vi "ViChoice.vi"() -> ()   [LabVIEW 2015]
uses:
  GlobalPath.vi
  GlobalVi.vi
  GlobalData.vi
panel:
  out "Finalization":bool
  out "Lines":string[](array[string])
  out "PinInsertGlue":bool
  out "QAQCvacoff":bool
  out "StiffRemoval":bool
  out "QAQCvacon":bool
  out "DrunRunFull":bool
  out "AllCoolBar":bool
  out "AddHoneycomb":bool
  out "AddFrame":bool
  out "PCBalignStiff":bool
  out "PCBposStiff":bool
  out "PCBalignTab":bool
  out "NewPanel":bool
  in  "Construction Finalization":bool
  in  "Panel QA/QC vacuum off":bool
  in  "Gluing of alignment pin/insert":bool
  in  "Panel QA/QC vacuum on":bool
  in  "Stiffback removal":bool
  in  "Add Cooling Bars":bool
  in  "Add Honeycomb":bool
  in  "Add Frames":bool
  in  "Dry Run (full)":bool
  in  "PCB Alignment on stiffback":bool
  in  "PCB Positioning on stiffback":bool
  in  "PCB Alignment on table":bool
  in  "New Panel":bool
  in  "current vi path":path
  out "Opening program":string
  in  "PCB gluing on table":bool
  in  "Internal structure positioning":bool
  in  "Stiffback gluing":bool
  in  "PCB Positioning on table":bool
  in  "Panel Closure":bool
  out "closePanel":bool
  out "PCBposTab":bool
  out "stbackPCBglue":bool
  out "tablePCBglue":bool
  out "innerStructure":bool
  # "Status"
  # "Control"
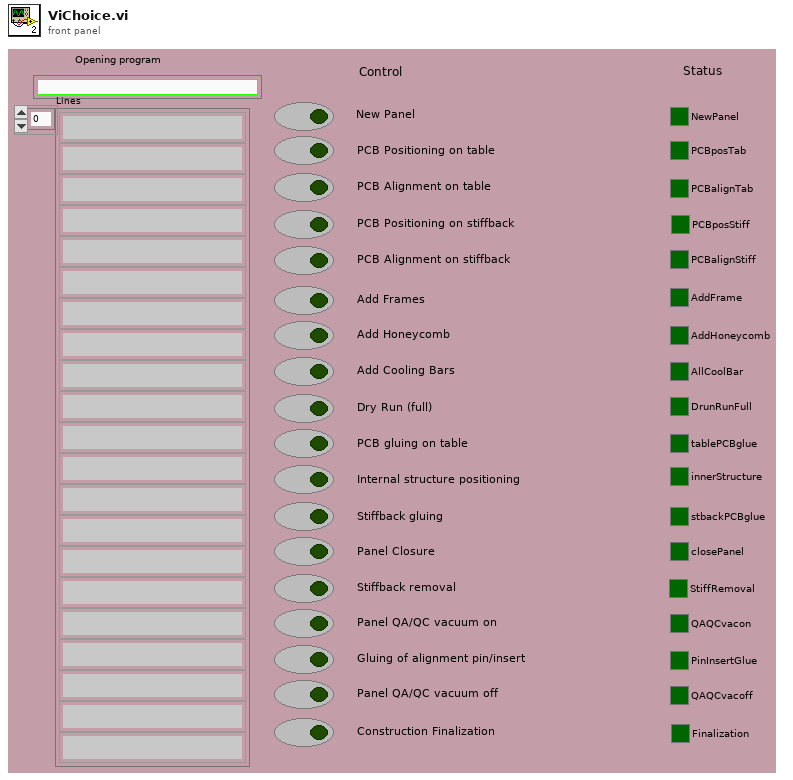
[diagram p1: front panel]
types:
  T1 = enum16{"open", "replace", "create", "open or create", "replace or create", "replace or create with confirmation"}
  T2 = cluster{"top":i32, "left":i32, "bottom":i32, "right":i32}
  T3 = enum32{"Bad", "Idle", "Run top level", "Running"}
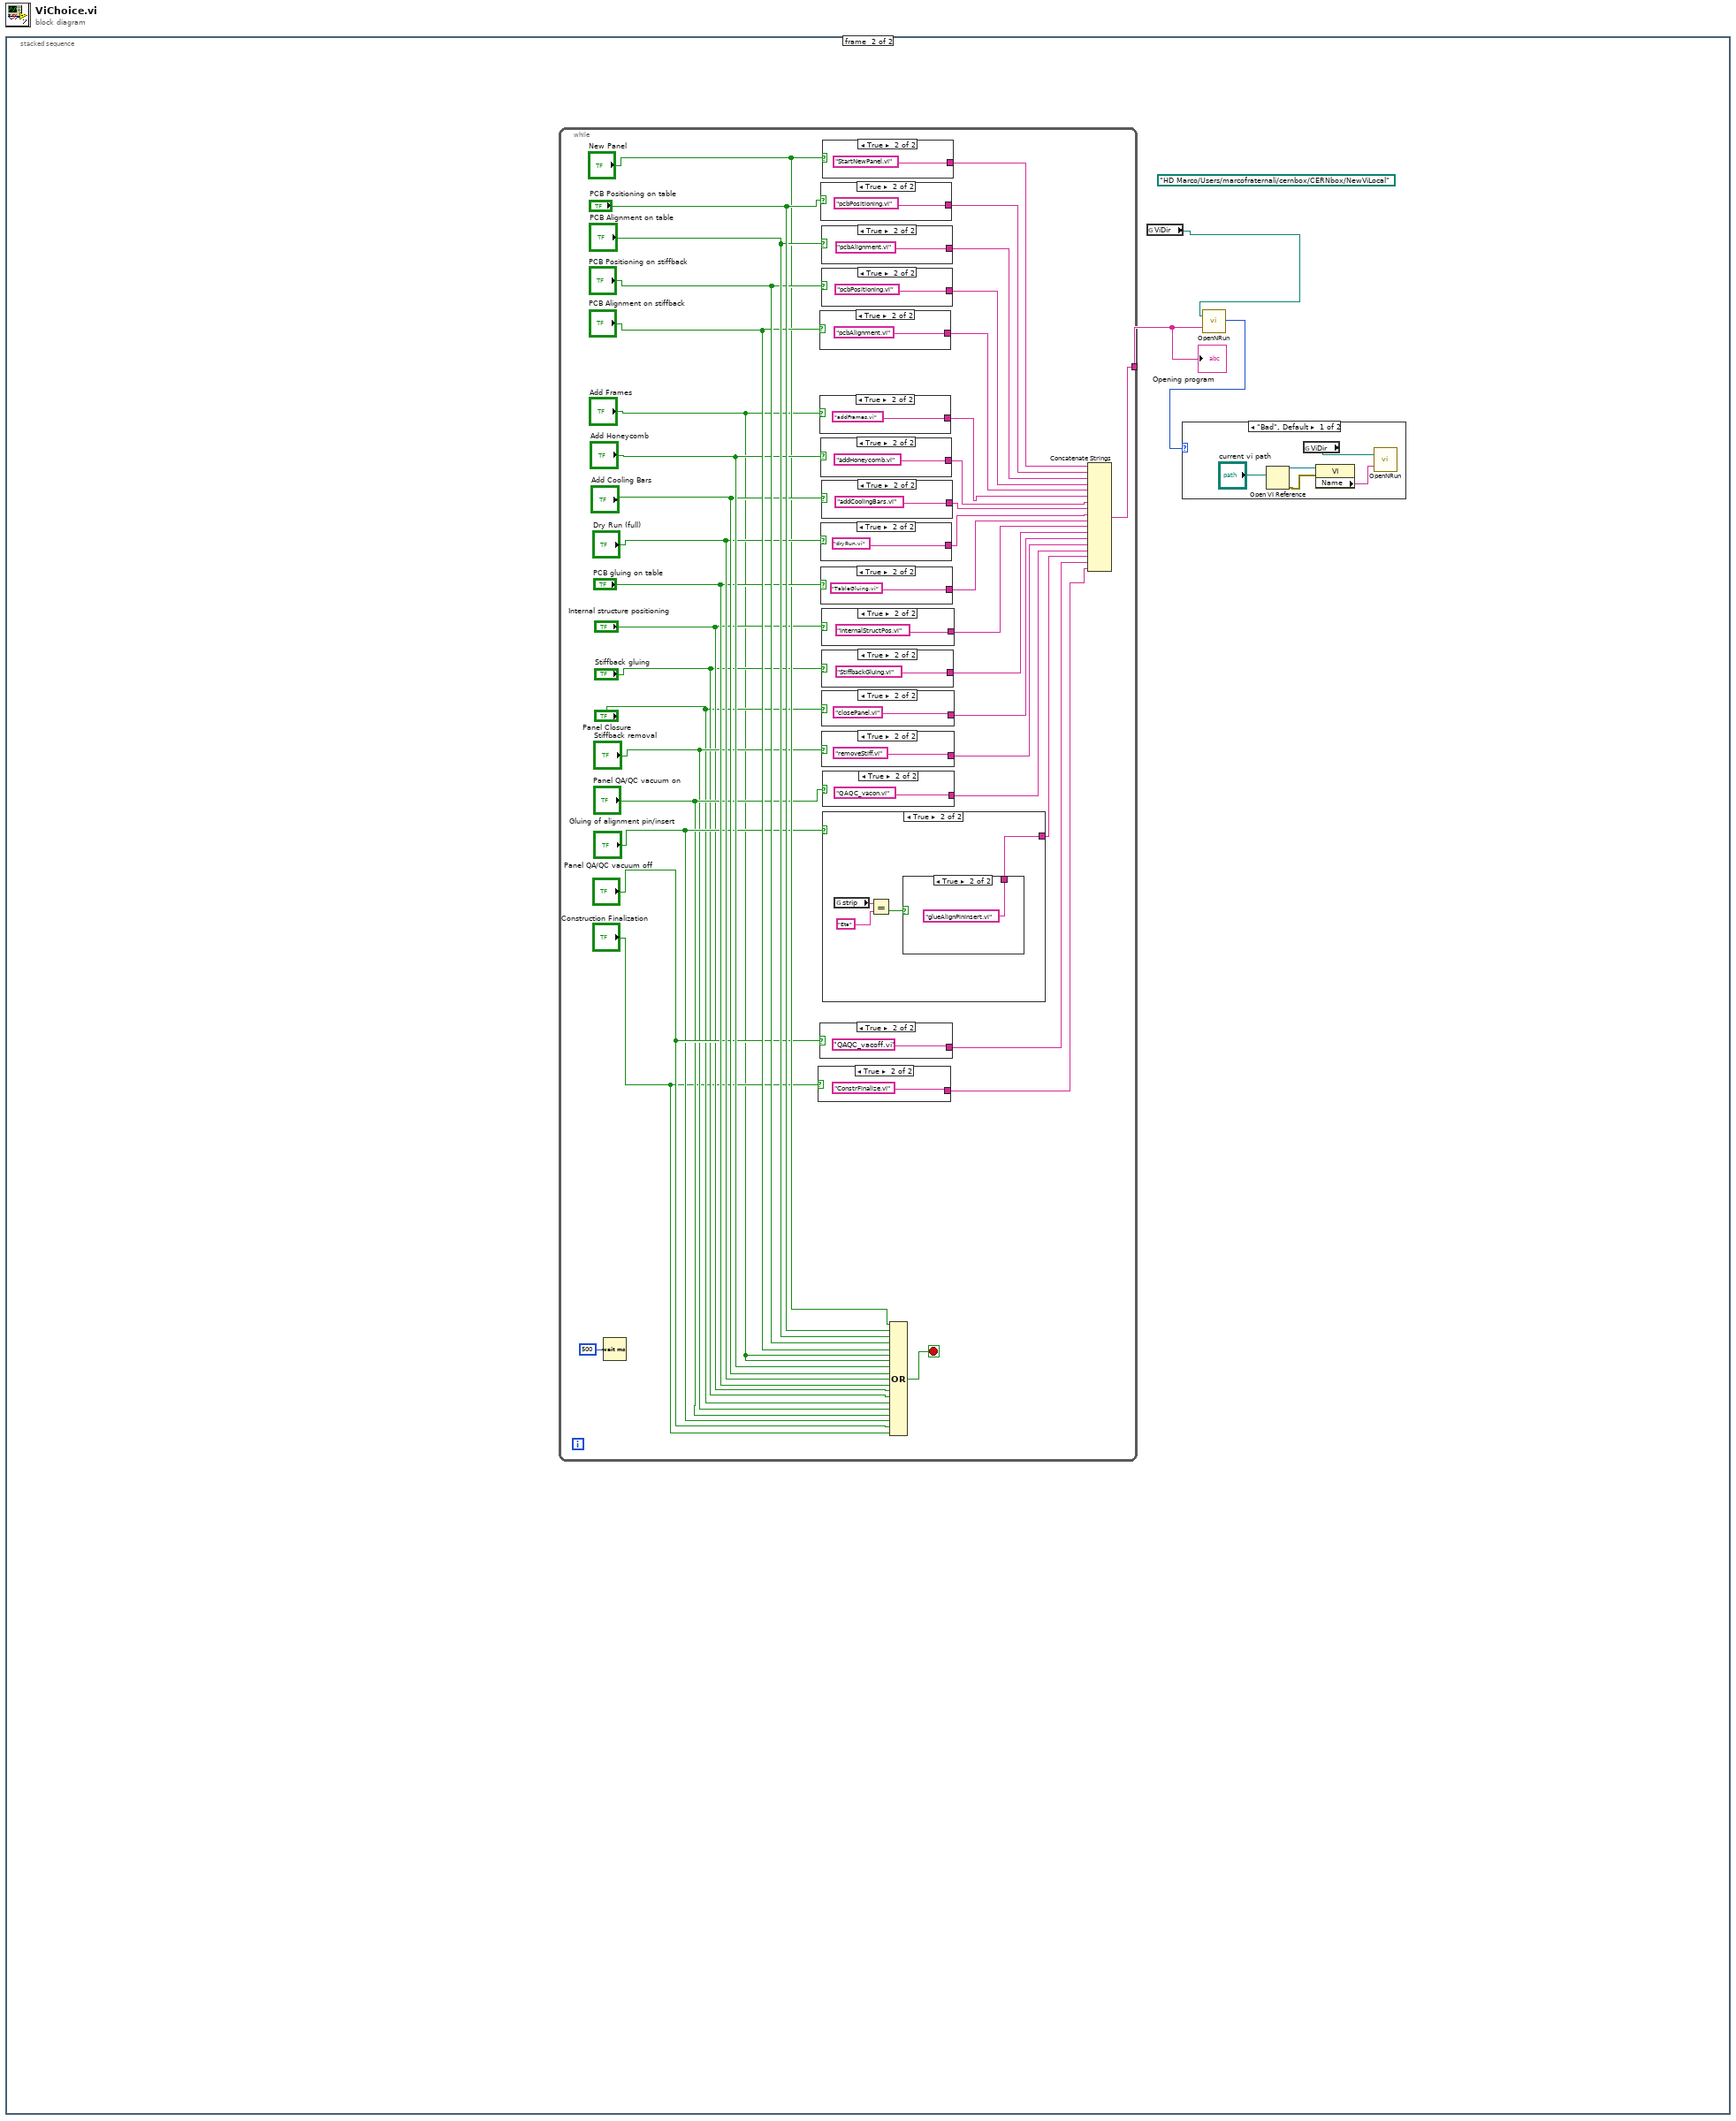
[diagram p0: block diagram]
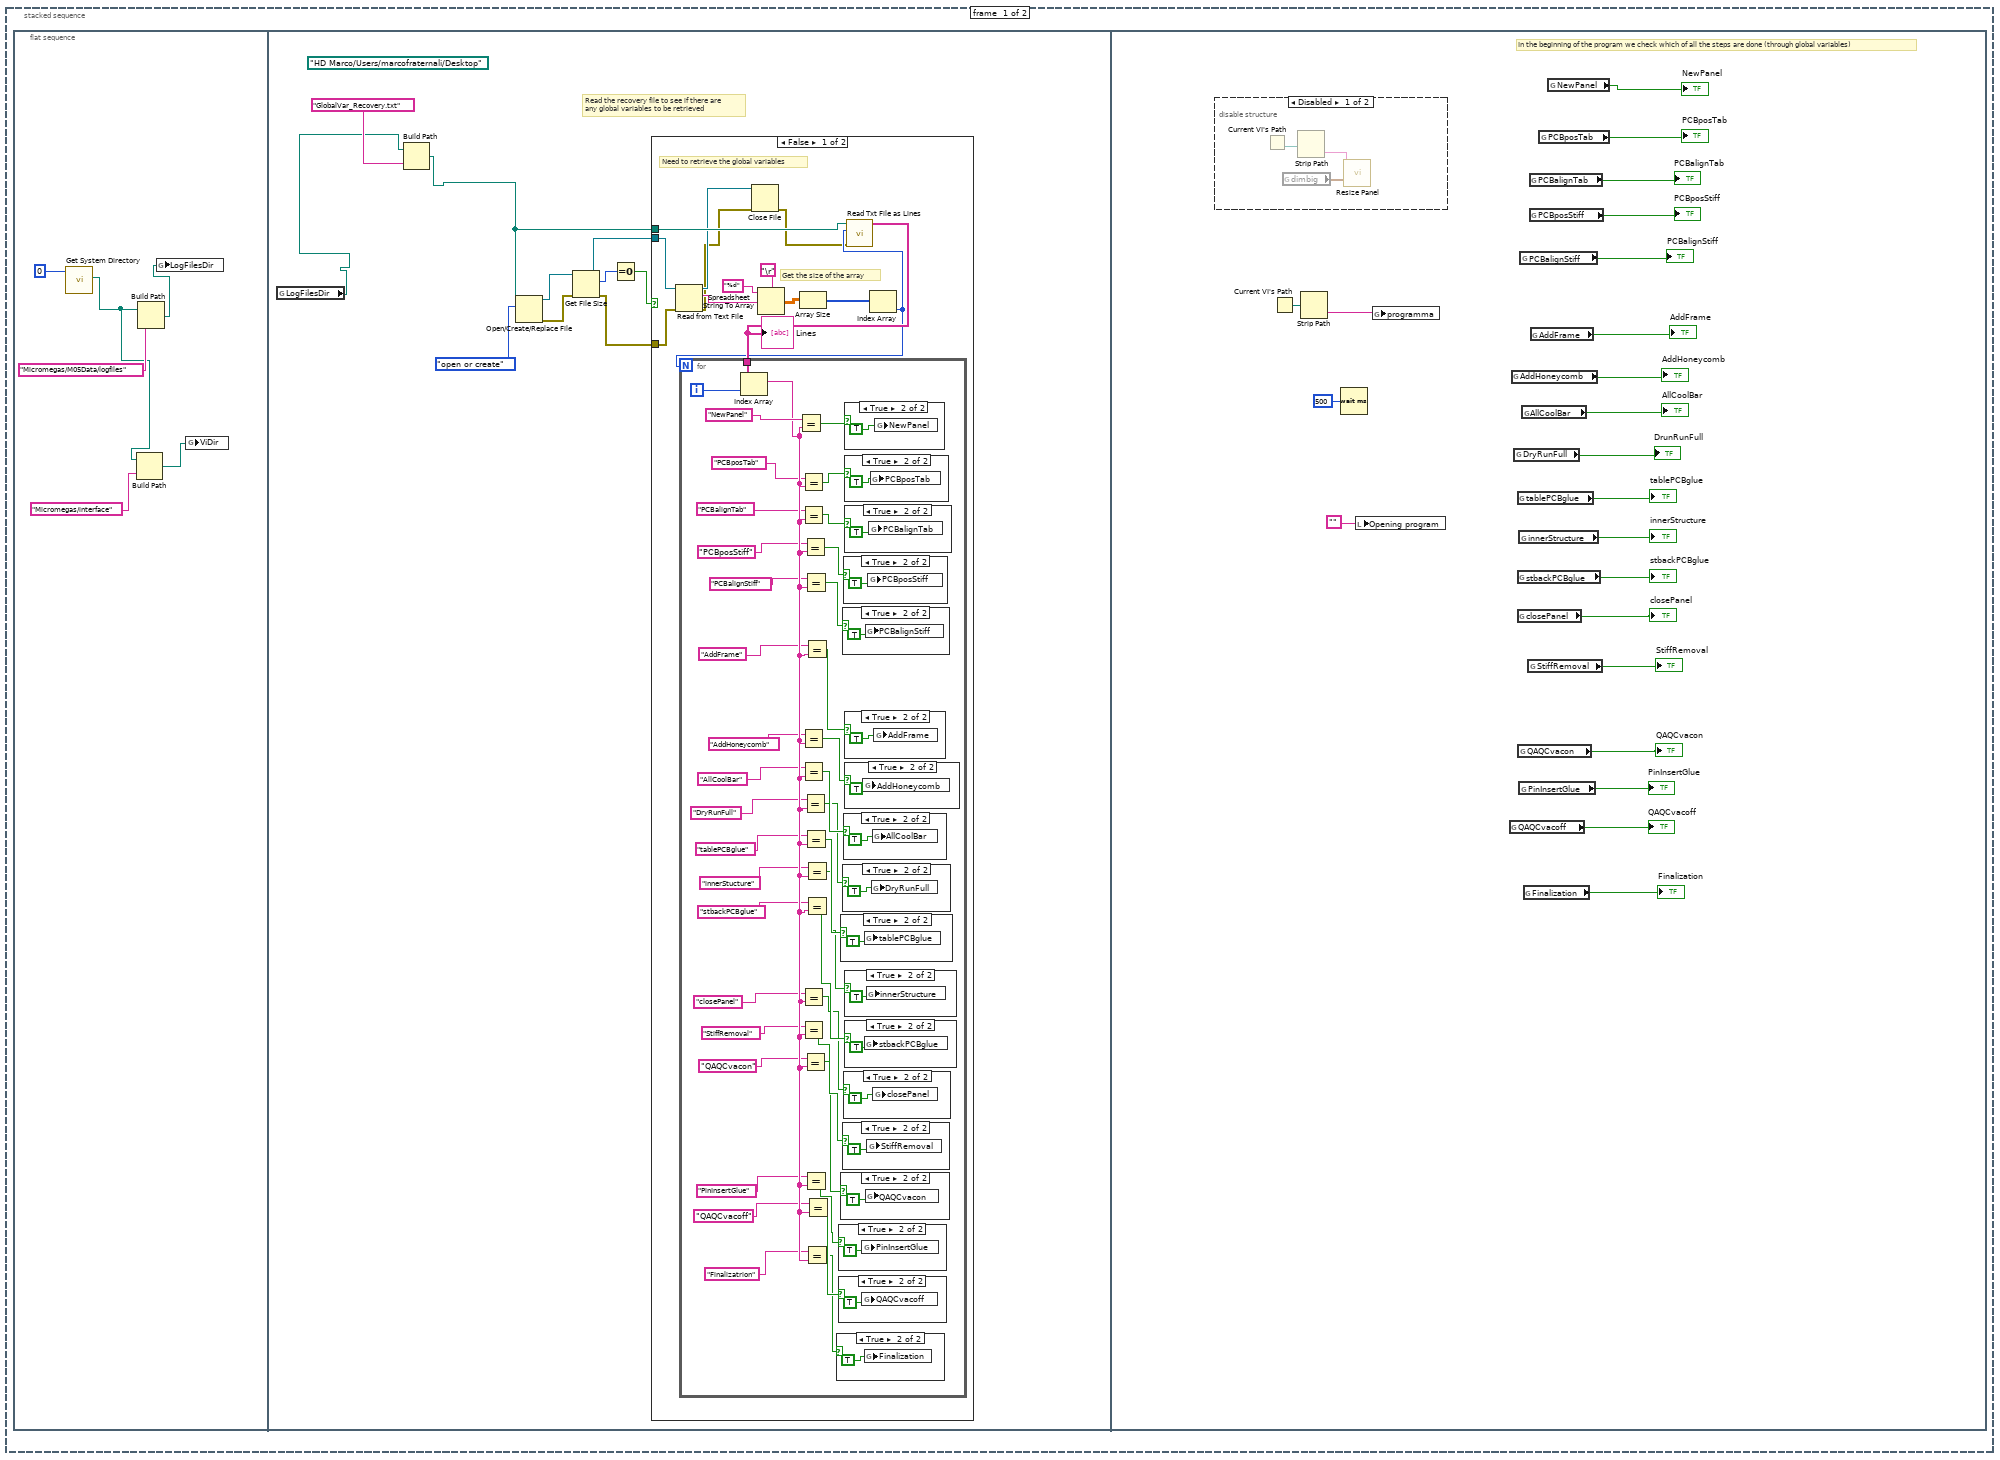
[diagram p2: hidden frame]
diagram:
  n1 = stacked-sequence {
    frame #0 {
      n2 = flat-sequence {
        frame #0 {
          n3 = call <vilib>:"Get System Directory.vi"("system directory type"=0) -> ("system directory"=w3:path)  [unwired: 10 in]
          n4 = Build Path(base path=w3, name or relative path="Micromegas/interface") -> (appended path=w2:path)
          n5 = Build Path(base path=w3, name or relative path="Micromegas/M05Data/logfiles") -> (appended path=w4:path)
          n6 = global write "GlobalPath.vi" "LogFilesDir"(w4) -> ()
          n7 = global write "GlobalPath.vi" "ViDir"(w2) -> ()
        }
        frame #1 {
          (unwired) path "/HD Marco/Users/marcofraternali/Desktop" ("path")
          # "Read the recovery file to see if there are\nany global variables to be retrieved"
          n8 = global read "GlobalPath.vi" "LogFilesDir"() -> (w7:path)
          n9 = Build Path(base path=w7, name or relative path="GlobalVar_Recovery.txt") -> (appended path=w8:path)
          n10 = Open/Create/Replace File(file path (use dialog)=w8, operation (0:open)=T1."open or create") -> (refnum out=w15:refnum<file>, error out=w13:errorcluster)  [unwired: 4 in, 1 out]
          n11 = Get File Size(file=w15, error in=w13) -> (refnum out=w11:refnum<file>, size (in bytes)=w14:i64, 0:w10:errorcluster)
          n12 = Equal To 0?(x=w14) -> (x = 0?=w12:bool)
          n13 = case shown="False" w12 {
            tunnel: w11 -> [w24 _]
            tunnel: w10 -> [w26 _]
            tunnel: w8 -> [w23 _]
            frame False {
              # "Get the size of the array"
              # "Need to retrieve the global variables"
              n14 = Read from Text File(file (use dialog)=w24, error in=w26) -> (refnum out=w19:refnum<file>, text=w27:string, error out=w18:errorcluster)  [unwired: 3 out]
              n15 = Close File(refnum=w19, error in=w18) -> (error out=w17:errorcluster)  [unwired: 1 out]
              n16 = Spreadsheet String To Array(delimiter (Tab)="\r", format string="%d", spreadsheet string=w27) -> (array=w25:dbl[][])  [unwired: 1 out]
              n17 = Array Size(array=w25) -> (size(s)=w22:i32[])
              n18 = Index Array(array=w22) -> (element=w20:i32)  [unwired: 1 in]
              n19 = call "Read Txt File as Lines.vi"("error in"=w17, "Lines to Read"=w20, "file path (use dialog)"=w23) -> ("Lines"=w21:string[])  [unwired: 7 in, 1 out]
              "Lines" <- w21
              n20 = for {
                N: w20 -> [_]
                tunnel: w21 -> [w68]
                i -> [w32]
                n21 = Index Array(array=w68, index=w32) -> (element=w49:string)
                n22 = Equal?(x="NewPanel", y=w49) -> (x = y?=w67:bool)
                n23 = Equal?(x="PCBposTab", y=w49) -> (x = y?=w66:bool)
                n24 = Equal?(x="PCBalignTab", y=w49) -> (x = y?=w65:bool)
                n25 = Equal?(x="AddHoneycomb", y=w49) -> (x = y?=w61:bool)
                n26 = Equal?(x="AllCoolBar", y=w49) -> (x = y?=w60:bool)
                n27 = Equal?(x="closePanel", y=w49) -> (x = y?=w55:bool)
                n28 = Equal?(x="StiffRemoval", y=w49) -> (x = y?=w54:bool)
                n29 = Equal?(x="PCBposStiff", y=w49) -> (x = y?=w64:bool)
                n30 = Equal?(x="DryRunFull", y=w49) -> (x = y?=w59:bool)
                n31 = Equal?(x="QAQCvacon", y=w49) -> (x = y?=w53:bool)
                n32 = Equal?(x="PCBalignStiff", y=w49) -> (x = y?=w63:bool)
                n33 = Equal?(x="tablePCBglue", y=w49) -> (x = y?=w58:bool)
                n34 = Equal?(x="PinInsertGlue", y=w49) -> (x = y?=w52:bool)
                n35 = Equal?(x="AddFrame", y=w49) -> (x = y?=w62:bool)
                n36 = Equal?(x="innerStucture", y=w49) -> (x = y?=w57:bool)
                n37 = Equal?(x="stbackPCBglue", y=w49) -> (x = y?=w56:bool)
                n38 = Equal?(x="Finalizatrion", y=w49) -> (x = y?=w30:bool)
                n39 = Equal?(x="QAQCvacoff", y=w49) -> (x = y?=w51:bool)
                n40 = case shown="True" w30 {
                  frame False {
                  }
                  frame True {
                    n41 = global write "GlobalVi.vi" "Finalization"(TRUE) -> ()
                  }
                }
                n42 = case shown="True" w52 {
                  frame False {
                  }
                  frame True {
                    n43 = global write "GlobalVi.vi" "PinInsertGlue"(TRUE) -> ()
                  }
                }
                n44 = case shown="True" w51 {
                  frame False {
                  }
                  frame True {
                    n45 = global write "GlobalVi.vi" "QAQCvacoff"(TRUE) -> ()
                  }
                }
                n46 = case shown="True" w58 {
                  frame False {
                  }
                  frame True {
                    n47 = global write "GlobalVi.vi" "tablePCBglue"(TRUE) -> ()
                  }
                }
                n48 = case shown="True" w53 {
                  frame False {
                  }
                  frame True {
                    n49 = global write "GlobalVi.vi" "QAQCvacon"(TRUE) -> ()
                  }
                }
                n50 = case shown="True" w63 {
                  frame False {
                  }
                  frame True {
                    n51 = global write "GlobalVi.vi" "PCBalignStiff"(TRUE) -> ()
                  }
                }
                n52 = case shown="True" w59 {
                  frame False {
                  }
                  frame True {
                    n53 = global write "GlobalVi.vi" "DryRunFull"(TRUE) -> ()
                  }
                }
                n54 = case shown="True" w54 {
                  frame False {
                  }
                  frame True {
                    n55 = global write "GlobalVi.vi" "StiffRemoval"(TRUE) -> ()
                  }
                }
                n56 = case shown="True" w64 {
                  frame False {
                  }
                  frame True {
                    n57 = global write "GlobalVi.vi" "PCBposStiff"(TRUE) -> ()
                  }
                }
                n58 = case shown="True" w60 {
                  frame False {
                  }
                  frame True {
                    n59 = global write "GlobalVi.vi" "AllCoolBar"(TRUE) -> ()
                  }
                }
                n60 = case shown="True" w55 {
                  frame False {
                  }
                  frame True {
                    n61 = global write "GlobalVi.vi" "closePanel"(TRUE) -> ()
                  }
                }
                n62 = case shown="True" w67 {
                  frame False {
                  }
                  frame True {
                    n63 = global write "GlobalVi.vi" "NewPanel"(TRUE) -> ()
                  }
                }
                n64 = case shown="True" w66 {
                  frame False {
                  }
                  frame True {
                    n65 = global write "GlobalVi.vi" "PCBposTab"(TRUE) -> ()
                  }
                }
                n66 = case shown="True" w65 {
                  frame False {
                  }
                  frame True {
                    n67 = global write "GlobalVi.vi" "PCBalignTab"(TRUE) -> ()
                  }
                }
                n68 = case shown="True" w62 {
                  frame False {
                  }
                  frame True {
                    n69 = global write "GlobalVi.vi" "AddFrame"(TRUE) -> ()
                  }
                }
                n70 = case shown="True" w61 {
                  frame False {
                  }
                  frame True {
                    n71 = global write "GlobalVi.vi" "AddHoneycomb"(TRUE) -> ()
                  }
                }
                n72 = case shown="True" w57 {
                  frame False {
                  }
                  frame True {
                    n73 = global write "GlobalVi.vi" "innerStructure"(TRUE) -> ()
                  }
                }
                n74 = case shown="True" w56 {
                  frame False {
                  }
                  frame True {
                    n75 = global write "GlobalVi.vi" "stbackPCBglue"(TRUE) -> ()
                  }
                }
              }
            }
            frame True {
              # "File is empty so nothing to retrieve"
            }
          }
        }
        frame #2 {
          # "In the beginning of the program we check which of all the steps are done (through global variables)"
          n76 = disable-structure shown="Disabled" {
            frame Disabled {
              n77 = Current VI's Path() -> (path=w111:path)
              n78 = global read "GlobalVi.vi" "dimbig"() -> (w109:T2)
              n79 = Strip Path(path=w111) -> (name=w110:string)  [unwired: 1 out]
              n80 = call <vilib>:"Resize Panel.vi"("panel location and size"=w109, "VI name"=w110) -> ()  [unwired: 9 in, 1 out]
            }
            frame Enabled {
            }
          }
          n81 = Current VI's Path() -> (path=w108:path)
          n82 = Strip Path(path=w108) -> (name=w100:string)  [unwired: 1 out]
          n83 = Wait (ms)(milliseconds to wait=u32 500) -> ()  [unwired: 1 out]
          n84 = local write "Opening program"("") -> ()
          n85 = global write "GlobalData.vi" "programma"(w100) -> ()
          n86 = global read "GlobalVi.vi" "QAQCvacoff"() -> (→"QAQCvacoff":bool)
          n87 = global read "GlobalVi.vi" "AddHoneycomb"() -> (→"AddHoneycomb":bool)
          n88 = global read "GlobalVi.vi" "DryRunFull"() -> (→"DrunRunFull":bool)
          n89 = global read "GlobalVi.vi" "tablePCBglue"() -> (→"tablePCBglue":bool)
          n90 = global read "GlobalVi.vi" "stbackPCBglue"() -> (→"stbackPCBglue":bool)
          n91 = global read "GlobalVi.vi" "closePanel"() -> (→"closePanel":bool)
          n92 = global read "GlobalVi.vi" "QAQCvacon"() -> (→"QAQCvacon":bool)
          n93 = global read "GlobalVi.vi" "innerStructure"() -> (→"innerStructure":bool)
          n94 = global read "GlobalVi.vi" "PinInsertGlue"() -> (→"PinInsertGlue":bool)
          n95 = global read "GlobalVi.vi" "PCBalignStiff"() -> (→"PCBalignStiff":bool)
          n96 = global read "GlobalVi.vi" "AllCoolBar"() -> (→"AllCoolBar":bool)
          n97 = global read "GlobalVi.vi" "Finalization"() -> (→"Finalization":bool)
          n98 = global read "GlobalVi.vi" "StiffRemoval"() -> (→"StiffRemoval":bool)
          n99 = global read "GlobalVi.vi" "PCBalignTab"() -> (→"PCBalignTab":bool)
          n100 = global read "GlobalVi.vi" "PCBposStiff"() -> (→"PCBposStiff":bool)
          n101 = global read "GlobalVi.vi" "AddFrame"() -> (→"AddFrame":bool)
          n102 = global read "GlobalVi.vi" "PCBposTab"() -> (→"PCBposTab":bool)
          n103 = global read "GlobalVi.vi" "NewPanel"() -> (→"NewPanel":bool)
        }
      }
    }
    frame #1 {
      (unwired) path "/HD Marco/Users/marcofraternali/cernbox/CERNbox/NewViLocal" ("path")
      n104 = while {
        tunnel: [w158] -> w114
        stop <- w159 stop-if-true
        n105 = Wait (ms)(milliseconds to wait=u32 500) -> ()  [unwired: 1 out]
        n106 = case shown="True" "Construction Finalization" {
          tunnel: ["" "ConstrFinalize.vi"] -> w122
          frame False {
          }
          frame True {
          }
        }
        n107 = case shown="True" "PCB Alignment on stiffback" {
          tunnel: ["" "pcbAlignment.vi"] -> w153
          frame False {
          }
          frame True {
          }
        }
        n108 = case shown="True" "Add Frames" {
          tunnel: ["" "addFrames.vi"] -> w135
          frame False {
          }
          frame True {
          }
        }
        n109 = case shown="True" "Panel QA/QC vacuum off" {
          tunnel: ["" "QAQC_vacoff.vi"] -> w123
          frame False {
          }
          frame True {
          }
        }
        n110 = case shown="True" "PCB Positioning on table" {
          tunnel: ["" "pcbPositioning.vi"] -> w157
          frame False {
          }
          frame True {
          }
        }
        n111 = case shown="True" "Add Honeycomb" {
          tunnel: ["" "addHoneycomb.vi"] -> w133
          frame False {
          }
          frame True {
          }
        }
        n112 = case shown="True" "Dry Run (full)" {
          tunnel: ["" "dryRun.vi"] -> w131
          frame False {
          }
          frame True {
          }
        }
        n113 = case shown="True" "PCB gluing on table" {
          tunnel: ["" "TableGluing.vi"] -> w130
          frame False {
          }
          frame True {
          }
        }
        n114 = case shown="True" "PCB Alignment on table" {
          tunnel: ["" "pcbAlignment.vi"] -> w155
          frame False {
          }
          frame True {
          }
        }
        n115 = case shown="True" "PCB Positioning on stiffback" {
          tunnel: ["" "pcbPositioning.vi"] -> w154
          frame False {
          }
          frame True {
          }
        }
        n116 = case shown="True" "Add Cooling Bars" {
          tunnel: ["" "addCoolingBars.vi"] -> w132
          frame False {
          }
          frame True {
          }
        }
        n117 = case shown="True" "Internal structure positioning" {
          tunnel: ["" "InternalStructPos.vi"] -> w129
          frame False {
          }
          frame True {
          }
        }
        n118 = case shown="True" "Stiffback gluing" {
          tunnel: ["" "StiffbackGluing.vi"] -> w128
          frame False {
          }
          frame True {
          }
        }
        n119 = case shown="True" "Panel Closure" {
          tunnel: ["" "closePanel.vi"] -> w127
          frame False {
          }
          frame True {
          }
        }
        n120 = case shown="True" "Stiffback removal" {
          tunnel: ["" "removeStiff.vi"] -> w126
          frame False {
          }
          frame True {
          }
        }
        n121 = case shown="True" "New Panel" {
          tunnel: ["" "StartNewPanel.vi"] -> w156
          frame False {
          }
          frame True {
          }
        }
        n122 = case shown="True" "Panel QA/QC vacuum on" {
          tunnel: ["" "QAQC_vacon.vi"] -> w125
          frame False {
          }
          frame True {
          }
        }
        n123 = case shown="True" "Gluing of alignment pin/insert" {
          tunnel: ["" w166] -> w124
          frame False {
          }
          frame True {
            n124 = global read "GlobalData.vi" "strip"() -> (w167:string)
            n125 = Equal?(x=w167, y="Eta") -> (x = y?=w169:bool)
            n126 = case shown="True" w169 {
              tunnel: ["glueAlignPinInsert_stereo.vi" "glueAlignPinInsert.vi"] -> w166
              frame False {
              }
              frame True {
              }
            }
          }
        }
        n127 = Compound Arithmetic op=OR("New Panel", "PCB Positioning on table", "PCB Alignment on table", "PCB Positioning on stiffback", "PCB Alignment on stiffback", "Add Frames", "Add Frames", "Add Honeycomb", "Add Cooling Bars", "Dry Run (full)", "PCB gluing on table", "Internal structure positioning", "Stiffback gluing", "Panel Closure", "Stiffback removal", "Panel QA/QC vacuum on", "Gluing of alignment pin/insert", "Panel QA/QC vacuum off", "Construction Finalization") -> (w159:bool)
        n128 = Concatenate Strings(w156, w157, w155, w154, w153, w135, w133, w132, w131, w130, w129, w128, w127, w126, w125, w124, w123, w122) -> (w158:string)
      }
      "Opening program" <- w114
      n129 = global read "GlobalPath.vi" "ViDir"() -> (w112:path)
      n130 = call "OpenNRun.vi"("VI name"=w114, "ViDirPath"=w112) -> ("Execution:State"=w113:T3)
      n131 = case shown="\"Bad\", Default" w113 {
        frame "Bad", Default {
          n132 = Open VI Reference(vi path="current vi path") -> (vi reference=w119:refnum<vi>, error out=w118:errorcluster)  [unwired: 5 in]
          n133 = global read "GlobalPath.vi" "ViDir"() -> (w116:path)
          n134 = property class="VI"(reference=w119, error in=w118) -> ("Name"=w115:string)  [unwired: 2 out]
          n135 = call "OpenNRun.vi"("VI name"=w115, "ViDirPath"=w116) -> ()  [unwired: 1 out]
        }
        frame "Idle" {
          n136 = Current VI's Path() -> (path=w120:path)
          n137 = Strip Path(path=w120) -> (name=w121:string)  [unwired: 1 out]
          n138 = call <vilib>:"Close Panel.vi"("VI name"=w121) -> ()  [unwired: 10 in, 1 out]
        }
      }
    }
  }
